vi "RT Driver VI.vi"(7 "Operation":T1, 11 "Device Reference in":T2 format="%.0x") -> (0 "Error Code":i32)   [LabVIEW 2019, in "J1939 Addon Engine.lvlib"]
uses:
  J1939 Addon Engine.lvlib
  <vilib>/NI VeriStand/Custom Device API/Custom Device Item Ref.ctl
  <vilib>/NI VeriStand/Custom Device API/Hardware Interface Driver VI Operation.ctl
  <vilib>/NI/NIVS Inline Async API/_VS Inline Async API/VS Inline Async API/Types/Error Handling Settings.ctl
  <vilib>/NI/NIVS Inline Async API/_VS Inline Async API/VS Inline Async API/VS Inline Async API.lvclass/VS Inline Async API.ctl
  <vilib>/NI/NIVS Inline Async API/_Data Access Engine/Data Access Engine/Data Access Engine.lvclass/Data Access Engine.ctl
  <vilib>/NI/NIVS Inline Async API/_Data Access Engine/Access Type Classes/Write/Write.lvclass/Write.ctl
  <vilib>/NI/NIVS Inline Async API/_Data Access Engine/Access Type Classes/ReadWrite/ReadWrite.lvclass/ReadWrite.ctl
  <vilib>/NI/NIVS Inline Async API/_Data Access Engine/Access Type Classes/Read/Read.lvclass/Read.ctl
  <vilib>/NI/NIVS Inline Async API/_Data Access Engine/Data Access Engine/Methods/Data.Engine.Read Data from HW.vi
  <vilib>/NI/NIVS Inline Async API/_VS Inline Async API/Error Handling Process/SubVIs/Error.GetError.vi
  <vilib>/NI VeriStand/Custom Device API/NI VeriStand - Set Channel Values by Block Data Reference.vi
  <vilib>/NI VeriStand/Custom Device API/NI VeriStand - Get Channel Values by Block Data Reference.vi
  <vilib>/NI/NIVS Inline Async API/_Data Access Engine/Data Access Engine/Methods/Data.Engine.Write Data to HW.vi
  <vilib>/NI/NIVS Inline Async API/_Data Access Engine/Access Type Classes/ReadWrite/ReadWrite.EngineData.vi
  <vilib>/NI/NIVS Inline Async API/_Data Access Engine/Access Type Classes/Write/Write.EngineData.vi
  <vilib>/NI/NIVS Inline Async API/_Data Access Engine/Access Type Classes/Read/Read.EngineData.vi
  <vilib>/NI VeriStand/Custom Device API/NI VeriStand - Get Channel Value by Data Reference.vi
  <vilib>/NI VeriStand/Custom Device API/NI VeriStand - Set Channel Value by Data Reference.vi
  <vilib>/Utility/SystemLogging/Write to System Log.vi
  SubVIs/Main.Load 986x Bitfile.vi
  SubVIs/Main.InitializeXNET.vi
  <vilib>/NI VeriStand/Custom Device API/Global Data Refs.vi
  <vilib>/xnet/xnet.llb/XNET Read.vi
  <vilib>/xnet/xnet.llb/XNET Read (Signal Single-point).vi
  <vilib>/xnet/xnet.llb/XNET Read (Signal XY).vi
  <vilib>/xnet/xnet.llb/XNET Write.vi
  <vilib>/xnet/xnet.llb/XNET Write (Signal Single-point).vi
  <vilib>/xnet/xnet.llb/XNET Stop.vi
  <vilib>/NI/NIVS Inline Async API/_VS Inline Async API/VS Inline Async API/VS Inline Async API.lvclass
  <vilib>/NI VeriStand/Custom Device API/Custom Device API.lvlib
  <vilib>/NI VeriStand/Custom Device Tools/Custom Device Utility Library/Custom Device Utility Library.lvlib
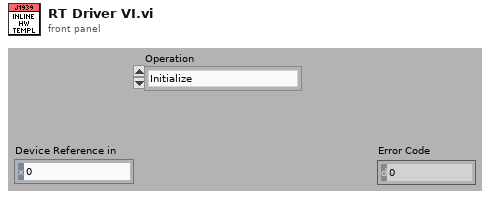
[diagram p1: front panel]
types:
  T1 = typedef "Custom Device API.lvlib/Hardware Interface Driver VI Operation.ctl" = enum16{"Initialize", "Start", "Read Data from HW", "Write Data to HW", "Close"}
  T2 = typedef "Custom Device API.lvlib/Custom Device Item Ref.ctl" = u64
  T3 = typedef "J1939 Addon Engine.lvlib/Main.State Variables.ctl" = cluster{"Main":T4, "Protocol":T5}
  T4 = typedef "J1939 Addon Engine.lvlib/Main.Settings.ctl" = cluster{"FPGA.Session":u32, "Incoming.Decimation":u32, "Outgoing.Decimation":u32, "Process":refnum<class "VS Inline Async API.lvclass">}
  T5 = typedef "J1939 Addon Engine.lvlib/Protocol.App Settings.ctl" = cluster{"Name":string, "XNET.Settings":T6, "Monitor.Network":T7, "Data":T8[], "DTCs":T20[], "Sim.Nodes.LUT":variant, "Data.LUT":variant, "PCL":u32}
  T6 = typedef "J1939 Addon Shared.lvlib/XNET Settings.ctl" = cluster{"Database":refnum<k21>, "Cluster":refnum<k21>, "Port":string, "Baud rate [Bd]":u32, "Termination":u32, "Incoming Decimation":u32, "Outgoing Decimation":u32}
  T7 = typedef "J1939 Addon Shared.lvlib/Monitor Settings.ctl" = cluster{"Address":u8, "Name":u64, "Include DA":bool}
  T8 = typedef "J1939 Addon Engine.lvlib/Protocol.XNET Refs.ctl" = cluster{"Network":T7, "Incoming.Use":bool, "Incoming.Session":refnum<k21>, "Incoming.Refs":T9[], "Incoming.Values":dbl[], "Outgoing.Frames":T11[], "Outgoing.Initialize":bool, "Outgoing.Refs":T9[], "Outgoing.Values":dbl[], "Request.Table":refnum<k33>, "Timing.Use":bool, "Timing.Index":i32[], "Timing.Refs":T9[], "Timing.Values":dbl[], "Disable.Refs":T9[], "Disable.Values":dbl[], "Trigger.Refs":T9[], "Trigger.Values":dbl[], "Outgoing.Frames.CountersAndProtections":T13[]}
  T9 = typedef "Custom Device API.lvlib/Block Data Reference.ctl" = cluster{"Data Reference":T10, "Offset":u64, "Length":u64}
  T10 = typedef "Custom Device API.lvlib/Data Reference.ctl" = i32
  T11 = typedef "J1939 Addon Engine.lvlib/Main.Outgoing.Frame.Settings.ctl" = cluster{"Offset":u32, "Length":u32, "Cyclic":bool, "Disable.Index":i32, "Disable":bool, "Trigger":T12, "Trigger.Index":i32, "Session":refnum<k21>}
  T12 = typedef "J1939 Addon Shared.lvlib/Outgoing Event Trigger Types.ctl" = enum16{"Channel value change", "Trigger channel (not zero)", "Channel value change or trigger channel (not zero)", "Trigger channel (any value change)", "Channel value change or trigger channel (any value change)"}
  T13 = typedef "Protection and Counter Support Shared.lvlib/Exported Frame Settings.ctl" = cluster{"Type":T14, "Frame ID":u32, "Payload Length":u32, "Signal XNET Paths":string[], "Frame.PrevData":dbl[], "VS Offset":i32, "VS Length":i32, "Generation Period":u32, "Has Protection?":bool, "Protection Configurations":T15[], "Has Counter":bool, "Counter Configurations":T18[], "Has Disable?":bool, "Disable VS Index":i32, "Transmit Trigger":T19, "Trigger VS Index":i32}
  T14 = typedef "Protection and Counter Support Shared.lvlib/Exported Frame Type.ctl" = enum16{"Periodic", "Event", "Periodic/Event"}
  T15 = typedef "Protection and Counter Support Shared.lvlib/Exported Protection Settings.ctl" = cluster{"Protection Frame Index":i32, "Protection Type":T16, "Data Indeces":i32[], "Initialized Data Array":dbl[], "Protection Signal XNET Paths":string[], "CRC Channels":T17[], "Protection VS Update Index":i32}
  T16 = typedef "Protection and Counter Support Shared.lvlib/Protection Type.ctl" = enum16{"Arb ID + Bytes Checksum with Inversion", "Arb ID + Bytes CRC with Inversion", "Reversed Raw Signal Checksum with Inversion", "Concatenated Two's Compliment"}
  T17 = typedef "Protection and Counter Support Shared.lvlib/XNET Signal Configuration.ctl" = cluster{"Start Bit":i32, "Name":string, "Number of bits":i32, "Scale":dbl, "Offset":dbl, "Data Type":u32, "Counter":bool}
  T18 = typedef "Protection and Counter Support Shared.lvlib/Exported Counter Settings.ctl" = cluster{"Frame Index":i32, "Max Count":dbl, "VS Index":i32, "Bit Length":i64}
  T19 = typedef "Protection and Counter Support Shared.lvlib/Exported Event Trigger Type.ctl" = enum16{"Channel value change", "Trigger channel (not zero)", "Channel value change or trigger channel (not zero)", "Trigger channel (any value change)", "Channel value change or trigger channel (any value change)"}
  T20 = typedef "J1939 Addon Engine.lvlib/Engine.DTC Settings.ctl" = cluster{"Data":T21, "FIFOs":T22}
  T21 = typedef "J1939 Addon Shared.lvlib/Compiled Simulated Settings.ctl" = cluster{"DM1.Ref":T9[], "DM1.Value":dbl[], "DM1.Enable.Ref":T9[], "DM1.Enable.Value":dbl[], "DM2.Ref":T9[], "DM2.Value":dbl[], "DM2.Enable.Ref":T9[], "DM2.Enable.Value":dbl[]}
  T22 = typedef "J1939 Addon Engine.lvlib/Engine.DTC FIFOs.ctl" = cluster{"DM1.Data":refnum<k33>, "DM1.Enable":refnum<k33>, "DM2.Data":refnum<k33>, "DM2.Enable":refnum<k33>, "DM1.Reset":refnum<k33>, "DM2.Reset":refnum<k33>}
  T23 = typedef "VS Inline Async API.lvlib/VS Inline Async API.lvclass/Error Handling Settings.ctl" = cluster{"Write to SystemLog (F)":bool}
  T24 = typedef "J1939 Addon Shared.lvlib/Compile Addon Settings.ctl" = cluster{"XNET":T6, "Bitfile":T25, "Nodes":T26, "Name":string}
  T25 = typedef "J1939 Addon Shared.lvlib/SysDef FPGA Settings.ctl" = cluster{"RT Path":path, "RIO Device":string, "Enable":bool}
  T26 = typedef "J1939 Addon Shared.lvlib/Compiled.Node Settings.ctl" = cluster{"Monitor":T27, "Sim":T33[]}
  T27 = typedef "J1939 Addon Shared.lvlib/Compiled Monitor Tool Settings.ctl" = cluster{"Network":T7, "Data":T28}
  T28 = typedef "J1939 Addon Shared.lvlib/Device Settings.ctl" = cluster{"Incoming":T29, "Outgoing":T31}
  T29 = typedef "J1939 Addon Shared.lvlib/Incoming Settings.ctl" = cluster{"Signals":string[], "Frames":T30[], "Data.Refs":T9[], "Data.Values":dbl[], "Timing.Use":bool, "Timing.Refs":T9[], "Timing.Values":dbl[], "Timing.Index":i32[]}
  T30 = typedef "J1939 Addon Shared.lvlib/Incoming Frame Settings.ctl" = cluster{"Signals":string[], "PGN":u32}
  T31 = typedef "J1939 Addon Shared.lvlib/Outgoing Settings.ctl" = cluster{"Frames":T32[], "Data.Refs":T9[], "Data.Values":dbl[], "Disable.Refs":T9[], "Disable.Values":dbl[], "Trigger.Refs":T9[], "Trigger.Values":dbl[], "Frames.CountersAndProtections":T13[]}
  T32 = typedef "J1939 Addon Shared.lvlib/Outgoing Frame Settings.ctl" = cluster{"Signals":string[], "Channel Array Position":cluster{"Offset":u32, "Length":u32}, "PGN":u32, "Cyclic?":bool, "Disable?":bool, "Disable.Index":i32, "Trigger":T12, "Trigger.Index":i32}
  T33 = typedef "J1939 Addon Shared.lvlib/Complied Simulated Device Settings.ctl" = cluster{"Network":T7, "Data":T28, "DTCs":T21}
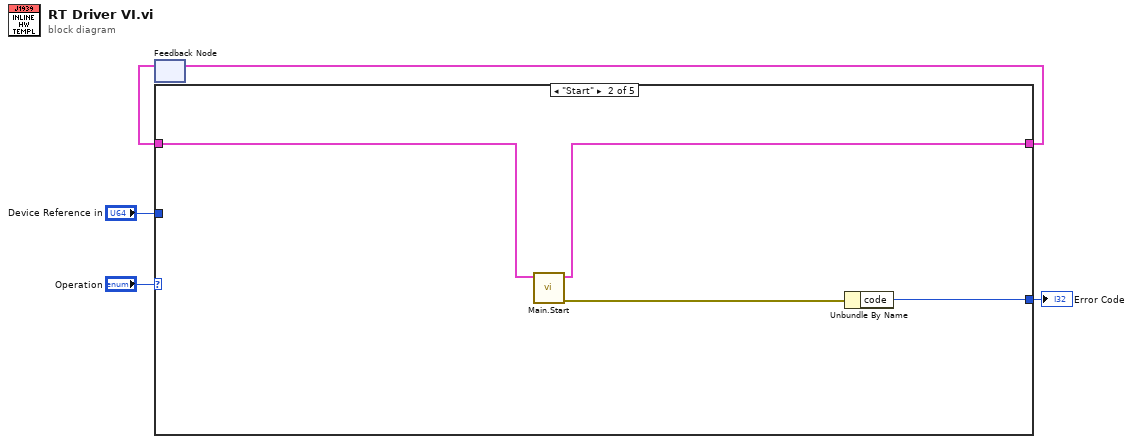
[diagram p0: block diagram]
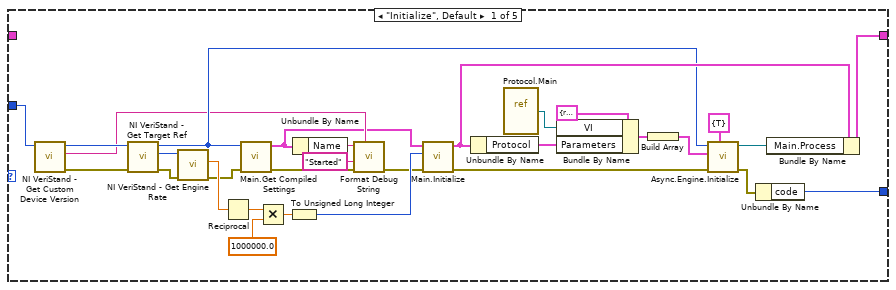
[diagram p2: hidden frame]
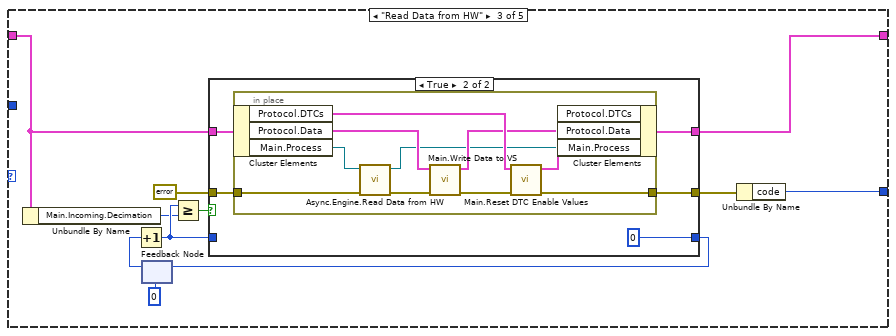
[diagram p3: hidden frame]
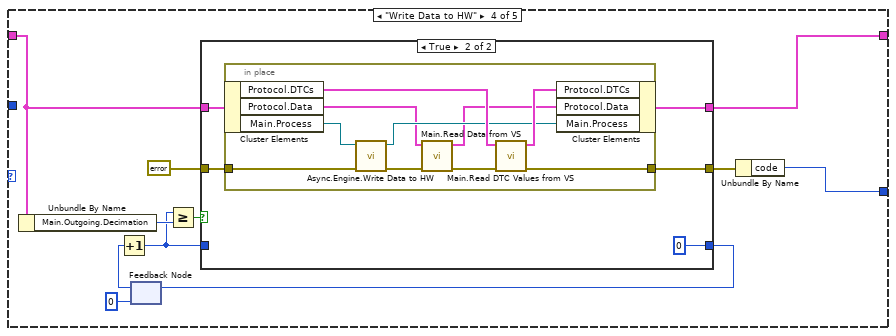
[diagram p5: hidden frame]
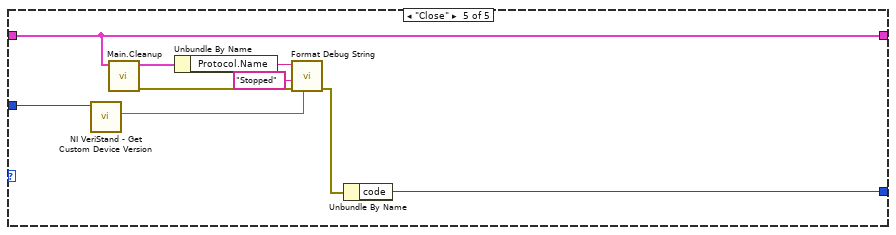
[diagram p7: hidden frame]
diagram:
  n1 = feedback #1() -> (w3:T3)  [unwired: 1 out]
  n2 = case shown="\"Start\"" "Operation" {
    tunnel: [w34 w38 w49 w79 w98] -> w4
    tunnel: w3 -> [_ w36 w50 w76 w98]
    tunnel: [w35 w39 w41 w70 w104] -> w2
    tunnel: "Device Reference in" -> [w33 _ _ _ w105]
    frame "Initialize", Default {
      n3 = call <vilib>:"NI VeriStand - Get Custom Device Version.vi"("Device Ref in"=w33) -> ("error out"=w16:errorcluster, "Value"=w10:string, "Device Ref out"=w18:T2)  [unwired: 8 in]
      n4 = call <vilib>:"NI VeriStand - Get Target Ref.vi"("error in"=w16, "Item Ref in"=w18) -> ("error out"=w15:errorcluster, "Target Ref"=w23:T2, "Item Ref out"=w17:T2)  [unwired: 6 in, 1 out]
      n5 = call <vilib>:"NI VeriStand - Get Engine Rate.vi"("error in (no error)"=w15, "Item Ref in"=w23) -> ("error out"=w14:errorcluster, "Rate (Hz)"=w22:dbl)  [unwired: 7 in, 1 out]
      n6 = Reciprocal(x=w22) -> (1/x=w21:dbl)
      n7 = call "Main.Get Compiled Settings.vi"("error in (no error)"=w14, "Item Ref in"=w17) -> ("error out"=w12:errorcluster, "Compiled"=w9:T24)  [unwired: 8 in]
      n8 = Multiply(x=w21, y=1000000.0) -> (x*y=w19:dbl)
      n9 = To Unsigned Long Integer(number=w19) -> (unsigned 32bit integer=w13:u32)
      n10 = Unbundle By Name(w9) -> ("Name"=w8:string)
      n11 = call "Format Debug String.vi"("Version"=w10, "error in (no error)"=w12, "State"="Started", "Name"=w8) -> ("error out"=w11:errorcluster)  [unwired: 7 in]
      n12 = call "Main.Initialize.vi"("error in (no error)"=w11, "PCL"=w13, "Compiled Settings"=w9) -> ("error out"=w32:errorcluster, "State Variables"=w25:T3)  [unwired: 7 in]
      n13 = Unbundle By Name(w25) -> ("Protocol"=w29:T5)
      n14 = vi-ref "Protocol.Main.vi"() -> (w26:refnum<vi>)
      n15 = Bundle By Name(cluster=cluster{"VI":refnum<vi>, "Parameters":variant} {"VI"=refnum, "Parameters"=variant} ("Process"), "VI"=w26, "Parameters"=w29) -> (w27:cluster{"VI":refnum<vi>, "Parameters":variant})
      n16 = Build Array(w27) -> (w24:cluster{"VI":refnum<vi>, "Parameters":variant}[])
      n17 = call <vilib>:"Async.Engine.Initialize.vi"("Error Log Settings"=T23 {"Write to SystemLog (F)"=TRUE}, "error in (no error)"=w32, "Processes"=w24, "Custom Device Ref"=w17) -> ("error out"=w31:errorcluster, "Async"=w30:refnum<class "VS Inline Async API.lvclass">)  [unwired: 6 in]
      n18 = Unbundle By Name(w31) -> ("code"=w35:i32)
      n19 = Bundle By Name(cluster=w25, "Main.Process"=w30) -> (w34:T3)
    }
    frame "Start" {
      n20 = call "Main.Start.vi"("State Variables in"=w36) -> ("error out"=w37:errorcluster, "State Variables out"=w38:T3)  [unwired: 9 in]
      n21 = Unbundle By Name(w37) -> ("code"=w39:i32)
    }
    frame "Read Data from HW" {
      n22 = Unbundle By Name(w50) -> ("Main.Incoming.Decimation"=w44:u32)
      n23 = feedback #2(u32 0) -> (w47:u32)
      n24 = Increment(x=w47) -> (x+1=w45:u32)
      n25 = Greater Or Equal?(x=w45, y=w44) -> (x >= y?=w46:bool)
      n26 = case shown="True" w46 {
        tunnel: w50 -> [w52 w57]
        tunnel: [w52 w56] -> w49
        tunnel: [w53 u32 0] -> w43
        tunnel: w45 -> [w53 _]
        tunnel: [w51 w55] -> w42
        tunnel: errorcluster {"status"=FALSE, "code"=0, "source"=""} ("error in (no error)") -> [w51 w54]
        frame False {
        }
        frame True {
          n27 = in-place {
            in-place-border: [w60] -> w55
            in-place-border: w54 -> [w59]
            n28 = in-place-cluster #3(w57) -> ("Protocol.DTCs"=w64:T20[], "Protocol.Data"=w65:T8[], "Main.Process"=w66:refnum<class "VS Inline Async API.lvclass">)
            n29 = call <vilib>:"Async.Engine.Read Data from HW.vi"("error in"=w59, "Async in"=w66) -> ("error out"=w68:errorcluster, "Async out"=w61:refnum<class "VS Inline Async API.lvclass">)  [unwired: 8 in]
            n30 = call "Main.Write Data to VS.vi"("error in"=w68, "Data Sessions"=w65) -> ("error out"=w67:errorcluster, "Data Sessions out"=w62:T8[])  [unwired: 8 in]
            n31 = call "Main.Reset DTC Enable Values.vi"("error in"=w67, "SimDTCs"=w64) -> ("error out"=w60:errorcluster, "SimDTCs"=w63:T20[])  [unwired: 8 in]
            n32 = in-place-cluster #3("Protocol.DTCs"=w63, "Protocol.Data"=w62, "Main.Process"=w61) -> (w56:T3)
          }
        }
      }
      n33 = feedback-in #2(w43) -> ()
      n34 = Unbundle By Name(w42) -> ("code"=w41:i32)
    }
    frame "Write Data to HW" {
      n35 = Unbundle By Name(w76) -> ("Main.Outgoing.Decimation"=w75:u32)
      n36 = feedback #4(u32 0) -> (w77:u32)
      n37 = Increment(x=w77) -> (x+1=w72:u32)
      n38 = Greater Or Equal?(x=w72, y=w75) -> (x >= y?=w74:bool)
      n39 = case shown="True" w74 {
        tunnel: w76 -> [w82 w86]
        tunnel: [w82 w85] -> w79
        tunnel: [w81 u32 0] -> w73
        tunnel: w72 -> [w81 _]
        tunnel: [w80 w84] -> w71
        tunnel: errorcluster {"status"=FALSE, "code"=0, "source"=""} ("error in (no error)") -> [w80 w83]
        frame False {
        }
        frame True {
          n40 = in-place {
            in-place-border: [w90] -> w84
            in-place-border: w83 -> [w88]
            n41 = in-place-cluster #5(w86) -> ("Protocol.DTCs"=w97:T20[], "Protocol.Data"=w93:T8[], "Main.Process"=w95:refnum<class "VS Inline Async API.lvclass">)
            n42 = call <vilib>:"Async.Engine.Write Data to HW.vi"("error in (no error)"=w88, "VS Inline Async API in"=w95) -> ("error out"=w89:errorcluster, "VS Inline Async API out"=w94:refnum<class "VS Inline Async API.lvclass">)  [unwired: 8 in]
            n43 = call "Main.Read Data from VS.vi"("error in"=w89, "Data Sessions"=w93) -> ("error out"=w91:errorcluster, "Data Sessions out"=w92:T8[])  [unwired: 8 in]
            n44 = call "Main.Read DTC Values from VS.vi"("error in"=w91, "Simulated Addresses in"=w97) -> ("error out"=w90:errorcluster, "Simulated Addresses out"=w96:T20[])  [unwired: 8 in]
            n45 = in-place-cluster #5("Protocol.DTCs"=w96, "Protocol.Data"=w92, "Main.Process"=w94) -> (w85:T3)
          }
        }
      }
      n46 = feedback-in #4(w73) -> ()
      n47 = Unbundle By Name(w71) -> ("code"=w70:i32)
    }
    frame "Close" {
      n48 = call <vilib>:"NI VeriStand - Get Custom Device Version.vi"("Device Ref in"=w105) -> ("Value"=w99:string)  [unwired: 8 in, 2 out]
      n49 = call "Main.Cleanup.vi"("State Variables"=w98) -> ("error out"=w101:errorcluster)  [unwired: 10 in]
      n50 = Unbundle By Name(w98) -> ("Protocol.Name"=w103:string)
      n51 = call "Format Debug String.vi"("Version"=w99, "error in (no error)"=w101, "State"="Stopped", "Name"=w103) -> ("error out"=w100:errorcluster)  [unwired: 7 in]
      n52 = Unbundle By Name(w100) -> ("code"=w104:i32)
    }
  }
  "Error Code" <- w2
  n53 = feedback-in #1(w4) -> ()
